vi "logging_get_parameter.vi"(5 "Error if not found (T)":bool=TRUE, 7 "Logging Parameter":T1, 8 "error in":errorcluster, 11 "Logging params in":variant) -> (0 "error out":errorcluster, 1 "String parameter out":string, 2 "I32 parameter out":i32, 3 "Logging params out":variant, 4 "Found":bool)   [LabVIEW 2014, in "rszvl_rsidr_core.lvlib"]
uses:
  rszvl_rsidr_core.lvlib
  type_Logging_Parameter.ctl
  type_Error_Codes.ctl
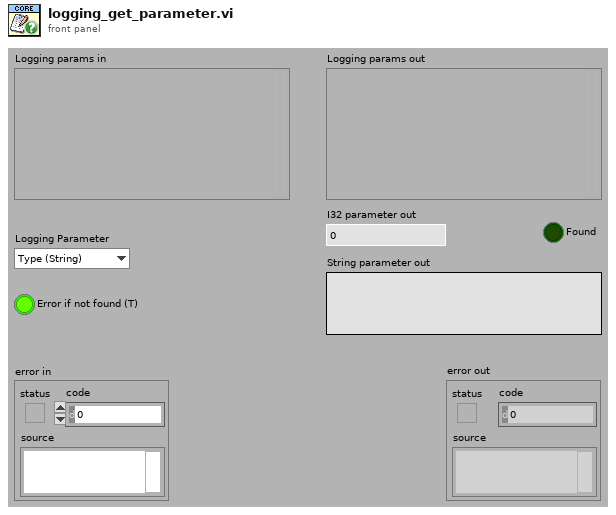
[diagram p1: front panel]
types:
  T1 = typedef "rszvl_rsidr_core.lvlib/type_Logging_Parameter.ctl" = enum16{"Type (String)", "SessionAlias(String)", "FormatString (String)", "UDPconectionID (I32)", "UDPlocalPort (I32)", "UDPremotePort (I32)", "UDPremoteHost (String)", "FILEmode (I32)", "FILEpath (String)", "FILEopenID (I32)"}
  T2 = typedef "rszvl_rsidr_core.lvlib/type_Error_Codes.ctl" = enum16{"No_error", "VISA_err_ResourceNotFound", "VISA_err_Timeout", "VISA_warn_MoreDataAvailable", "RS_err_MissingCallback", "RS_err_InvalidAttribute", "RS_err_InvalidValue", "RS_err_UnknownResource", "RS_err_AlreadyInitialized", "RS_err_InstrumentStatus", "RS_err_BadRepCapName", "RS_err_TypesMismatch", "RS_err_ValueNotSupported", "RS_err_InvalidRngTable", "RS_err_IDqueryFail", "RS_err_UnexpResponse", "VISA_warn_ConfigNotLoaded", "RS_err_AttributeNotReadable", "RS_err_AttributeNotWritable", "RS_err_InstrumentType", "RS_err_InstrumentOption", "VISA_err_InvalidSize", "RS_err_ReliabilityIndicator", "VISA_warn_UnknownStatus", "VISA_warn_TermCharRead", "VISA_err_IO_error"}
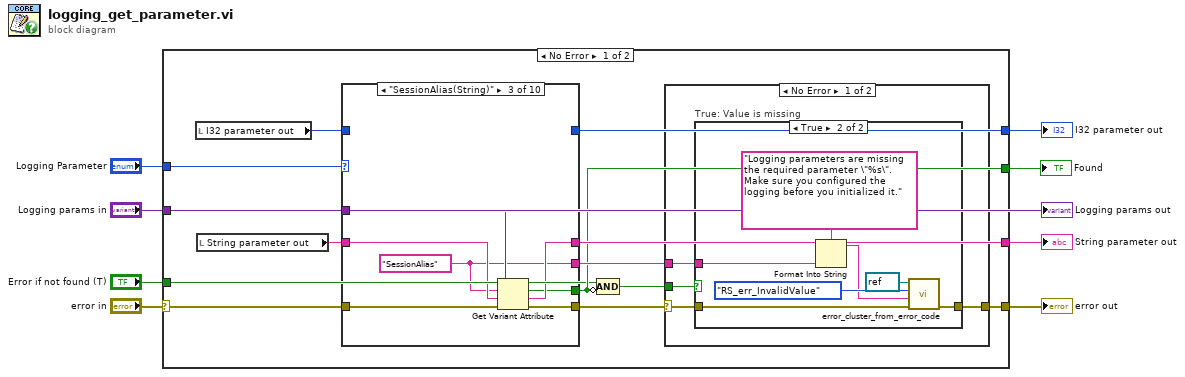
[diagram p0: block diagram]
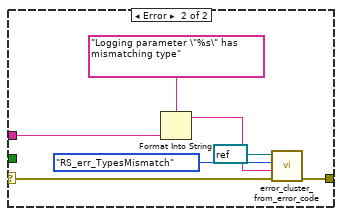
[diagram p3: hidden frame]
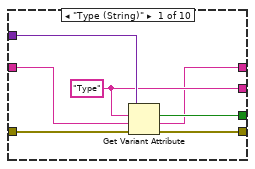
[diagram p4: hidden frame]
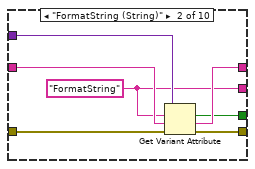
[diagram p5: hidden frame]
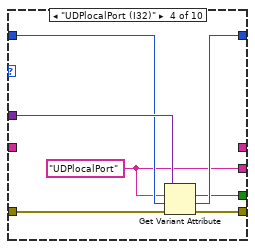
[diagram p6: hidden frame]
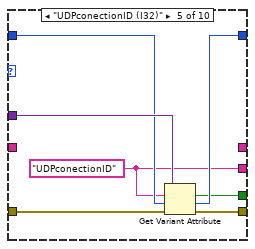
[diagram p7: hidden frame]
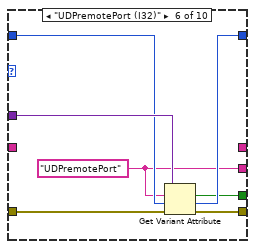
[diagram p8: hidden frame]
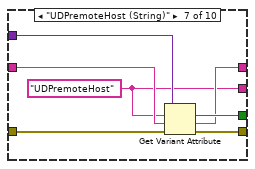
[diagram p9: hidden frame]
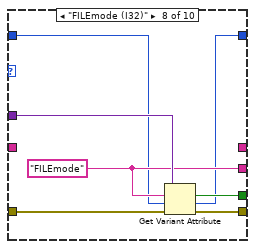
[diagram p10: hidden frame]
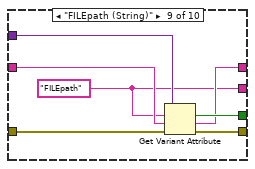
[diagram p11: hidden frame]
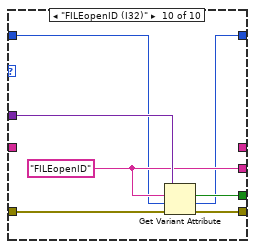
[diagram p12: hidden frame]
diagram:
  n1 = case shown="No Error" "error in" {
    selector: "error in" -> [w21 w111]
    tunnel: [w14 w111] -> w7
    tunnel: "Logging params in" -> [w20 _]
    tunnel: [w18 _] -> w6
    tunnel: [w17 _] -> w5
    tunnel: [w11 _] -> w3
    tunnel: "Error if not found (T)" -> [w10 _]
    tunnel: "Logging Parameter" -> [w9 _]
    frame No Error {
      n2 = local read "I32 parameter out"() -> (w19:i32)
      n3 = local read "String parameter out"() -> (w16:string)
      n4 = case shown="\"SessionAlias(String)\"" w9 {
        tunnel: w21 -> [w47 w54 w61 w68 w75 w82 w89 w96 w103 w110]
        tunnel: [w46 w53 w60 w67 w74 w81 w88 w95 w102 w109] -> w15
        tunnel: w20 -> [w45 w52 w59 w66 w73 w80 w87 w94 w101 w108]
        tunnel: w19 -> [_ _ _ w65 w72 w79 _ w90 _ w104]
        tunnel: w16 -> [w42 w51 w58 _ _ _ w86 _ w100 _]
        tunnel: [w41 w50 w57 _ _ _ w84 _ w98 _] -> w18
        tunnel: [_ _ _ w64 w71 w78 _ w91 _ w105] -> w17
        tunnel: [w44 w49 w56 w63 w70 w77 w85 w93 w99 w107] -> w11
        tunnel: [w43 w48 w55 w62 w69 w76 w83 w92 w97 w106] -> w13
        frame "Type (String)" {
          w43 = "Type"
          n5 = Get Variant Attribute(Variant=w45, name=w43, default value (empty Variant)=w42, error in=w47) -> (found=w44:bool, value=w41:string, error out=w46:errorcluster)  [unwired: 1 out]
        }
        frame "FormatString (String)" {
          w48 = "FormatString"
          n6 = Get Variant Attribute(Variant=w52, name=w48, default value (empty Variant)=w51, error in=w54) -> (found=w49:bool, value=w50:string, error out=w53:errorcluster)  [unwired: 1 out]
        }
        frame "SessionAlias(String)" {
          w55 = "SessionAlias"
          n7 = Get Variant Attribute(Variant=w59, name=w55, default value (empty Variant)=w58, error in=w61) -> (found=w56:bool, value=w57:string, error out=w60:errorcluster)  [unwired: 1 out]
        }
        frame "UDPlocalPort (I32)" {
          w62 = "UDPlocalPort"
          n8 = Get Variant Attribute(Variant=w66, name=w62, default value (empty Variant)=w65, error in=w68) -> (found=w63:bool, value=w64:i32, error out=w67:errorcluster)  [unwired: 1 out]
        }
        frame "UDPconectionID (I32)" {
          w69 = "UDPconectionID"
          n9 = Get Variant Attribute(Variant=w73, name=w69, default value (empty Variant)=w72, error in=w75) -> (found=w70:bool, value=w71:i32, error out=w74:errorcluster)  [unwired: 1 out]
        }
        frame "UDPremotePort (I32)" {
          w76 = "UDPremotePort"
          n10 = Get Variant Attribute(Variant=w80, name=w76, default value (empty Variant)=w79, error in=w82) -> (found=w77:bool, value=w78:i32, error out=w81:errorcluster)  [unwired: 1 out]
        }
        frame "UDPremoteHost (String)" {
          w83 = "UDPremoteHost"
          n11 = Get Variant Attribute(Variant=w87, name=w83, default value (empty Variant)=w86, error in=w89) -> (found=w85:bool, value=w84:string, error out=w88:errorcluster)  [unwired: 1 out]
        }
        frame "FILEmode (I32)" {
          w92 = "FILEmode"
          n12 = Get Variant Attribute(Variant=w94, name=w92, default value (empty Variant)=w90, error in=w96) -> (found=w93:bool, value=w91:i32, error out=w95:errorcluster)  [unwired: 1 out]
        }
        frame "FILEpath (String)" {
          w97 = "FILEpath"
          n13 = Get Variant Attribute(Variant=w101, name=w97, default value (empty Variant)=w100, error in=w103) -> (found=w99:bool, value=w98:string, error out=w102:errorcluster)  [unwired: 1 out]
        }
        frame "FILEopenID (I32)" {
          w106 = "FILEopenID"
          n14 = Get Variant Attribute(Variant=w108, name=w106, default value (empty Variant)=w104, error in=w110) -> (found=w107:bool, value=w105:i32, error out=w109:errorcluster)  [unwired: 1 out]
        }
      }
      n15 = Compound Arithmetic op=AND(w10, invert w11) -> (w12:bool)
      n16 = case shown="No Error" w15 {
        selector: w15 -> [w23 w39]
        tunnel: [w25 w40] -> w14
        tunnel: w13 -> [w24 w38]
        tunnel: w12 -> [w22 _]
        frame No Error {
          n17 = case "True: Value is missing" shown="True" w22 {
            tunnel: w23 -> [w26 w30]
            tunnel: [w26 w33] -> w25
            tunnel: w24 -> [_ w31]
            frame False {
            }
            frame True {
              n18 = Format Into String(format string="Logging parameters are missing the required parameter \"%s\". Make sure you configured the logging before you initialized it.", w31) -> (resulting string=w28:string)  [unwired: 2 in, 1 out]
              n19 = call "error_cluster_from_error_code.vi"("error in"=w30, "error message (\"\")"=w28, "Error Enum in"=type_Error_Codes."RS_err_InvalidValue", "VISA resource name"=refnum<visa-resource-name> refnum) -> ("error out"=w33:errorcluster)  [unwired: 6 in, 1 out]
            }
          }
        }
        frame Error {
          n20 = Format Into String(format string="Logging parameter \"%s\" has mismatching type", w38) -> (resulting string=w35:string)  [unwired: 2 in, 1 out]
          n21 = call "error_cluster_from_error_code.vi"("error in"=w39, "error message (\"\")"=w35, "Error Enum in"=type_Error_Codes."RS_err_TypesMismatch", "VISA resource name"=refnum<visa-resource-name> refnum) -> ("error out"=w40:errorcluster)  [unwired: 6 in, 1 out]
        }
      }
    }
    frame Error {
    }
  }
  "error out" <- w7
  "I32 parameter out" <- w5
  "String parameter out" <- w6
  "Found" <- w3
  "Logging params out" <- "Logging params in"
